vi "Clustered input func gen.vi"(9 "Settings":T1, 10 "beginning time":dbl, 11 "current time":dbl) -> (1 "finished?":bool, 2 "x-y output":cluster{"x":dbl, "y":dbl}, 4 "sample gap (ms)":dbl)   [LabVIEW 2013]
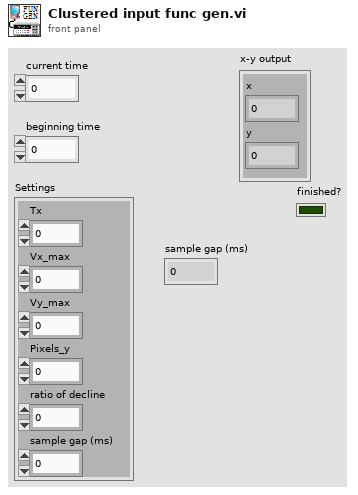
[diagram p1: front panel]
types:
  T1 = cluster{"Tx":dbl, "Vx_max":dbl, "Vy_max":dbl, "Pixels_y":i32, "ratio of decline":dbl, "sample gap (ms)":dbl}
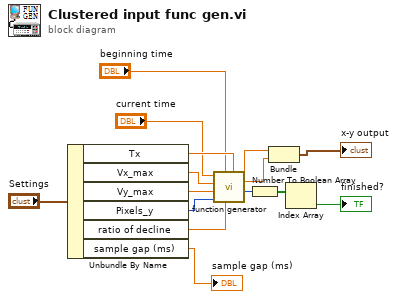
[diagram p0: block diagram]
diagram:
  n1 = Unbundle By Name("Settings") -> ("Tx"=w10:dbl, "Vx_max"=w11:dbl, "Vy_max"=w12:dbl, "Pixels_y"=w13:i32, "ratio of decline"=w14:dbl, "sample gap (ms)"=→"sample gap (ms)":dbl)
  n2 = call "function generator.vi"("Tx"=w10, "ratio of decline"=w14, "t_bgn"="beginning time", "Row_N"=w13, "Vy_max"=w12, "Vx_max"=w11, "t_cur"="current time") -> ("finished?"=w5:i32, "y"=w3:dbl, "x"=w4:dbl)  [unwired: 2 in]
  n3 = Number To Boolean Array(number=w5) -> (Boolean array=w6:bool[])
  n4 = Bundle("x"=w4, "y"=w3) -> (→"x-y output":cluster{"x":dbl, "y":dbl})  [unwired: 1 in]
  n5 = Index Array(array=w6) -> (element=→"finished?":bool)  [unwired: 1 in]
